vi "PC_COUNT_ALL_Stations_for_Year.vi"(0 "Refnum in":T1, 1 "data in":string[][](array[string]), 3 "Array 3":string[](array[string]), 5 "Select Year 2":string(combo), 7 "SHIFT":i32[](array[numeric]), 9 "STATION":i32[](array[numeric]), 11 "error in (no error)":errorcluster) -> (4 "Refnum out":T1, 6 "data out":string[][](array[string]), 8 "DATE":string[](array[string]), 10 "COUNT":string[](array[string]), 15 "error out":errorcluster)   [LabVIEW 2017]
uses:
  <vilib>/addons/database/Connection.llb/Conn ObjectReference.ctl
  <vilib>/addons/database/NI_Database_API.lvlib
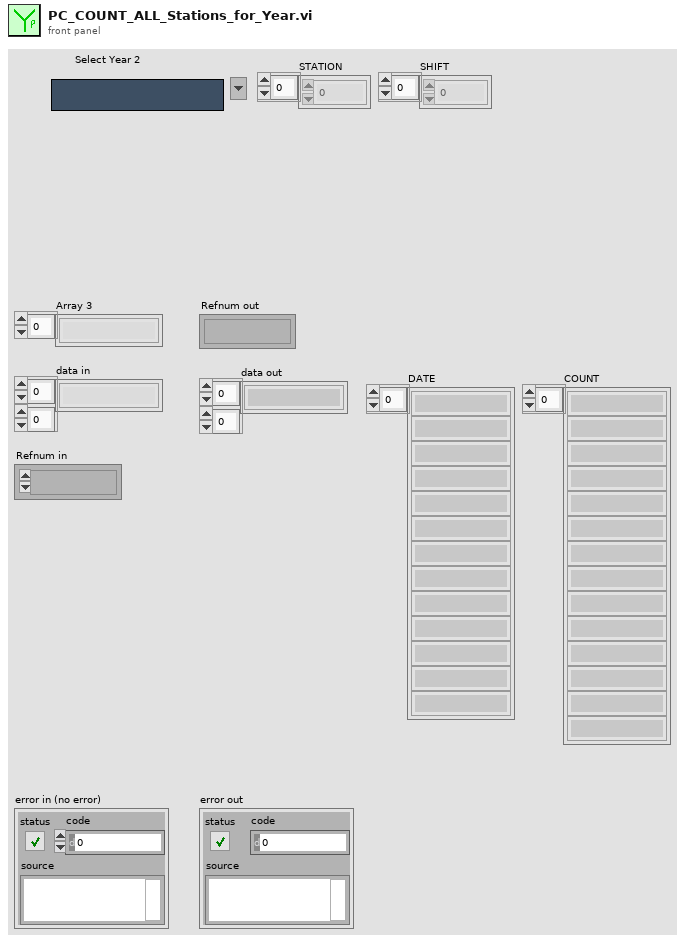
[diagram p1: front panel]
types:
  T1 = typedef "NI_Database_API.lvlib/Conn ObjectReference.ctl" = refnum<k1>
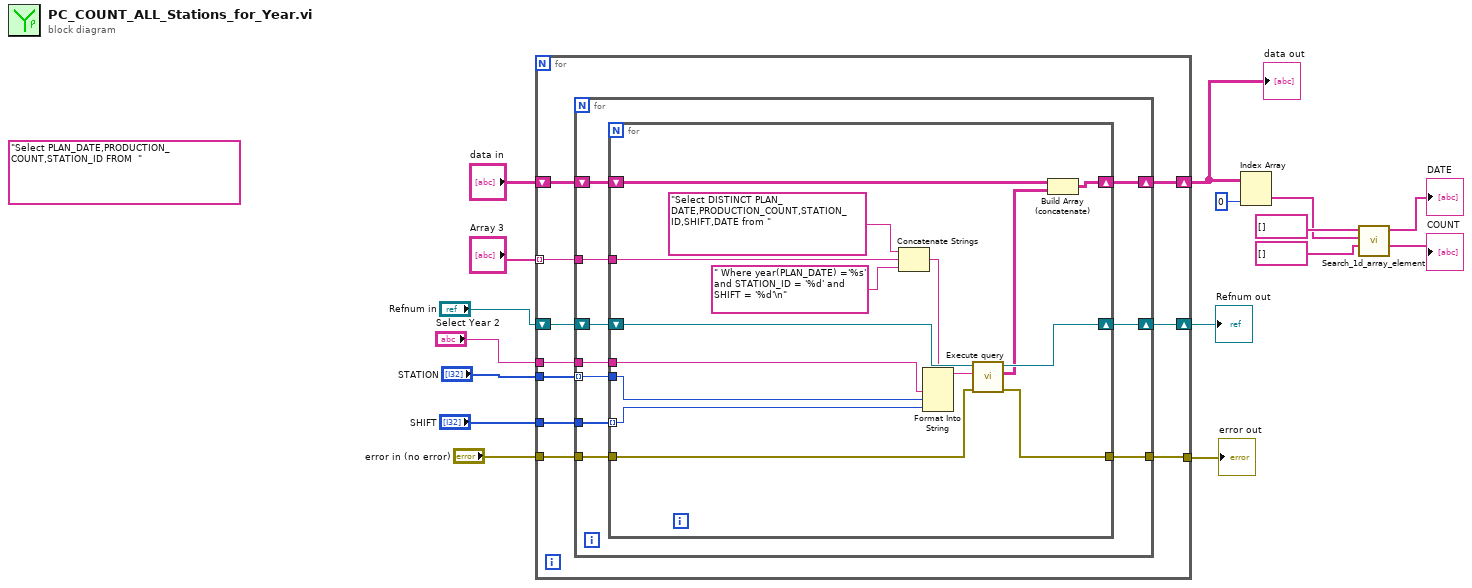
[diagram p0: block diagram]
diagram:
  (unwired) "Select PLAN_DATE,PRODUCTION_COUNT,STATION_ID FROM  "
  n1 = for {
    shift-right: [w25] -> w9
    shift-left: "Refnum in" -> [w26]
    tunnel: "Array 3" -> [w24] mode=indexing
    shift-right: [w20] -> w3
    shift-left: "data in" -> [w21]
    tunnel: "error in (no error)" -> [w23]
    tunnel: [w22] -> w13
    tunnel: "STATION" -> [w18]
    tunnel: "SHIFT" -> [w19]
    tunnel: "Select Year 2" -> [w17]
    n2 = for {
      tunnel: w24 -> [w34]
      tunnel: w19 -> [w29]
      shift-right: [w35] -> w25
      shift-left: w26 -> [w36]
      shift-right: [w30] -> w20
      shift-left: w21 -> [w31]
      tunnel: w18 -> [w28] mode=indexing
      tunnel: w23 -> [w33]
      tunnel: [w32] -> w22
      tunnel: w17 -> [w27]
      n3 = for {
        tunnel: w34 -> [w49]
        shift-right: [w50] -> w35
        shift-left: w36 -> [w51]
        shift-right: [w45] -> w30
        shift-left: w31 -> [w46]
        tunnel: w29 -> [w39] mode=indexing
        tunnel: w28 -> [w40]
        tunnel: w33 -> [w48]
        tunnel: [w47] -> w32
        tunnel: w27 -> [w37]
        n4 = Concatenate Strings("Select DISTINCT PLAN_DATE,PRODUCTION_COUNT,STATION_ID,SHIFT,DATE from ", w49, " Where year(PLAN_DATE) ='%s' and STATION_ID = '%d' and SHIFT = '%d'\n") -> (w43:string)
        n5 = Format Into String(format string=w43, w37, w40, w39) -> (resulting string=w44:string)  [unwired: 2 in, 1 out]
        n6 = call "Execute query.vi"("error in (no error)"=w48, "String"=w44, "connection reference"=w51) -> ("error out"=w47:errorcluster, "Table"=w41:string[][], "connection reference 2"=w50:T1)  [unwired: 5 in, 1 out]
        n7 = Build Array (concatenate)(w46, w41) -> (w45:string[][])
      }
    }
  }
  "data out" <- w3
  "error out" <- w13
  "Refnum out" <- w9
  n8 = Index Array(array=w3, index (col)=0 ("disabled index (col)")) -> (element=w6:string[])  [unwired: 1 in]
  n9 = call "Search_1d_array_element.vi"("Count in"=string[] [] ("Count"), "BD Date"=w6, "Elements Found in"=string[] [] ("Elements Found")) -> ("Count out"=→"COUNT":string[], "Elements Found out"=→"DATE":string[])  [unwired: 4 in, 1 out]
